vi "Display Command.vi"(8 "error in (no error)":errorcluster, 9 "Button Name":string, 10 "Command":string, 11 "First Actor in":refnum<class "First Actor.lvclass">) -> (0 "error out":errorcluster, 3 "First Actor out":refnum<class "First Actor.lvclass">)   [LabVIEW 2021, in "First Actor.lvlib" / "First Actor.lvclass"]
uses:
  First Actor.lvclass
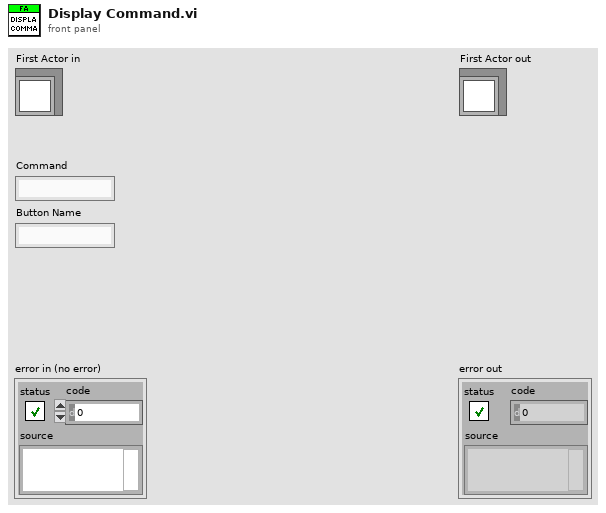
[diagram p1: front panel]
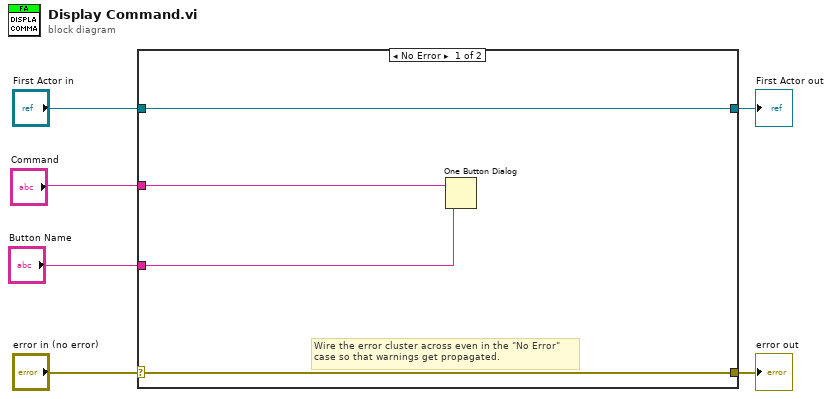
[diagram p0: block diagram]
diagram:
  n1 = case shown="No Error" "error in (no error)" {
    selector: "error in (no error)" -> [w9 w12]
    tunnel: [w9 w12] -> w5
    tunnel: [w10 w11] -> w3
    tunnel: "First Actor in" -> [w10 w11]
    tunnel: "Command" -> [w8 _]
    tunnel: "Button Name" -> [w7 _]
    frame No Error {
      # "Wire the error cluster across even in the \"No Error\"\ncase so that warnings get propagated."
      n2 = One Button Dialog(message=w8, button name ("OK")=w7) -> ()  [unwired: 1 out]
    }
    frame Error {
    }
  }
  "error out" <- w5
  "First Actor out" <- w3
